vi "ReadConfigurationFile_Algo(old).vi"(0 "Default Configuration file path":path=path "C:/Users/GTron/Desktop/MOTHERSON v1.3/ZenGage V1.3.1/Configuration file/Algorithm Parameters Default.json", 5 "Override Configuration file path":path=path "C:/Users/GTron/Desktop/MOTHERSON v1.3/ZenGage V1.3.1/Configuration file/Algorithm Parameters Override.json", 7 "OutputClusterIn":T1={"Acknowledgement"={"Enqueuer"=refnum, "VIReference"=refnum, "VIName"=""}, "AllPartInfo"=[{"PartName"="", "NumberOfRacks"=0, "MeasurementIDsArray"=[], "MeasurementNamesArray"=[], "SpecValuesArray"=[]}], "PartInfo"={"PartName"="", "TotalCount"=0, "ReelCount"=0, "NumberOfRacks"=0, "MeasurementIDsArray"=[], "MeasurementNamesArray"=[], "SpecValuesArray"=[]}, "Result Cluster"={"Measurement Names Array"=[], "Pass-Fail Array"=[], "Measurement Values Array "=[], "Roi for overlay (Arrows) Array"=[], "Algo Type Array"=[], "Image Array"=[], "Clamp operations"=enum."Average Clamp", "  Search Direction "=[], "Images_Array_in"=[], "ResultPF"=FALSE, "Total Cluster Values"={"Total Fail"=0, "Total Pass"=0, "Total Count"=0}, "Reel Counter Cluster"={"Reel Fail"=0, "Reel Pass"=0, "Reel Count"=0}, "Tolerance  Array"=[], "Array of Cam Spec Control Bool"=[], "Control Pass Fail Array"=[], "Specification Pass Fail Array"=[], "Overlay Arrow Lines"=[], "Camera ID"=[], "Trigger count"=0, "Specification fail?"=FALSE}}, 9 "AlgoParameters":T6, 11 "error in":errorcluster) -> (4 "OutputClusterOut":T1={"Acknowledgement"={"Enqueuer"=refnum, "VIReference"=refnum, "VIName"=""}, "AllPartInfo"=[], "PartInfo"={"PartName"="", "TotalCount"=0, "ReelCount"=0, "NumberOfRacks"=0, "MeasurementIDsArray"=[], "MeasurementNamesArray"=[], "SpecValuesArray"=[]}, "Result Cluster"={"Measurement Names Array"=[], "Pass-Fail Array"=[], "Measurement Values Array "=[], "Roi for overlay (Arrows) Array"=[], "Algo Type Array"=[], "Image Array"=[], "Clamp operations"=enum."Average Clamp", "  Search Direction "=[], "Images_Array_in"=[], "ResultPF"=FALSE, "Total Cluster Values"={"Total Fail"=0, "Total Pass"=0, "Total Count"=0}, "Reel Counter Cluster"={"Reel Fail"=0, "Reel Pass"=0, "Reel Count"=0}, "Tolerance  Array"=[], "Array of Cam Spec Control Bool"=[], "Control Pass Fail Array"=[], "Specification Pass Fail Array"=[], "Overlay Arrow Lines"=[], "Camera ID"=[], "Trigger count"=0, "Specification fail?"=FALSE}}, 6 "AllAlgoParameters":T6, 15 "error out":errorcluster)   [LabVIEW 2015, in "Algorithm.lvclass"]
uses:
  FrameworkOverrides/Algorithm.lvclass
  Controls/OutputCluster.ctl
  <vilib>/ActorFramework/Message Enqueuer/Message Enqueuer.lvclass
  Common/Controls/Acknowledgement.ctl
  Common/Controls/AllPartInfo.ctl
  Controls/Result Cluster.ctl
panel:
  out "Queried Cluster":variant
  out "Default JSON string":string
  out "Override JSON string":string
  out "Error Message":string
  out "Output Merged Cluster":variant
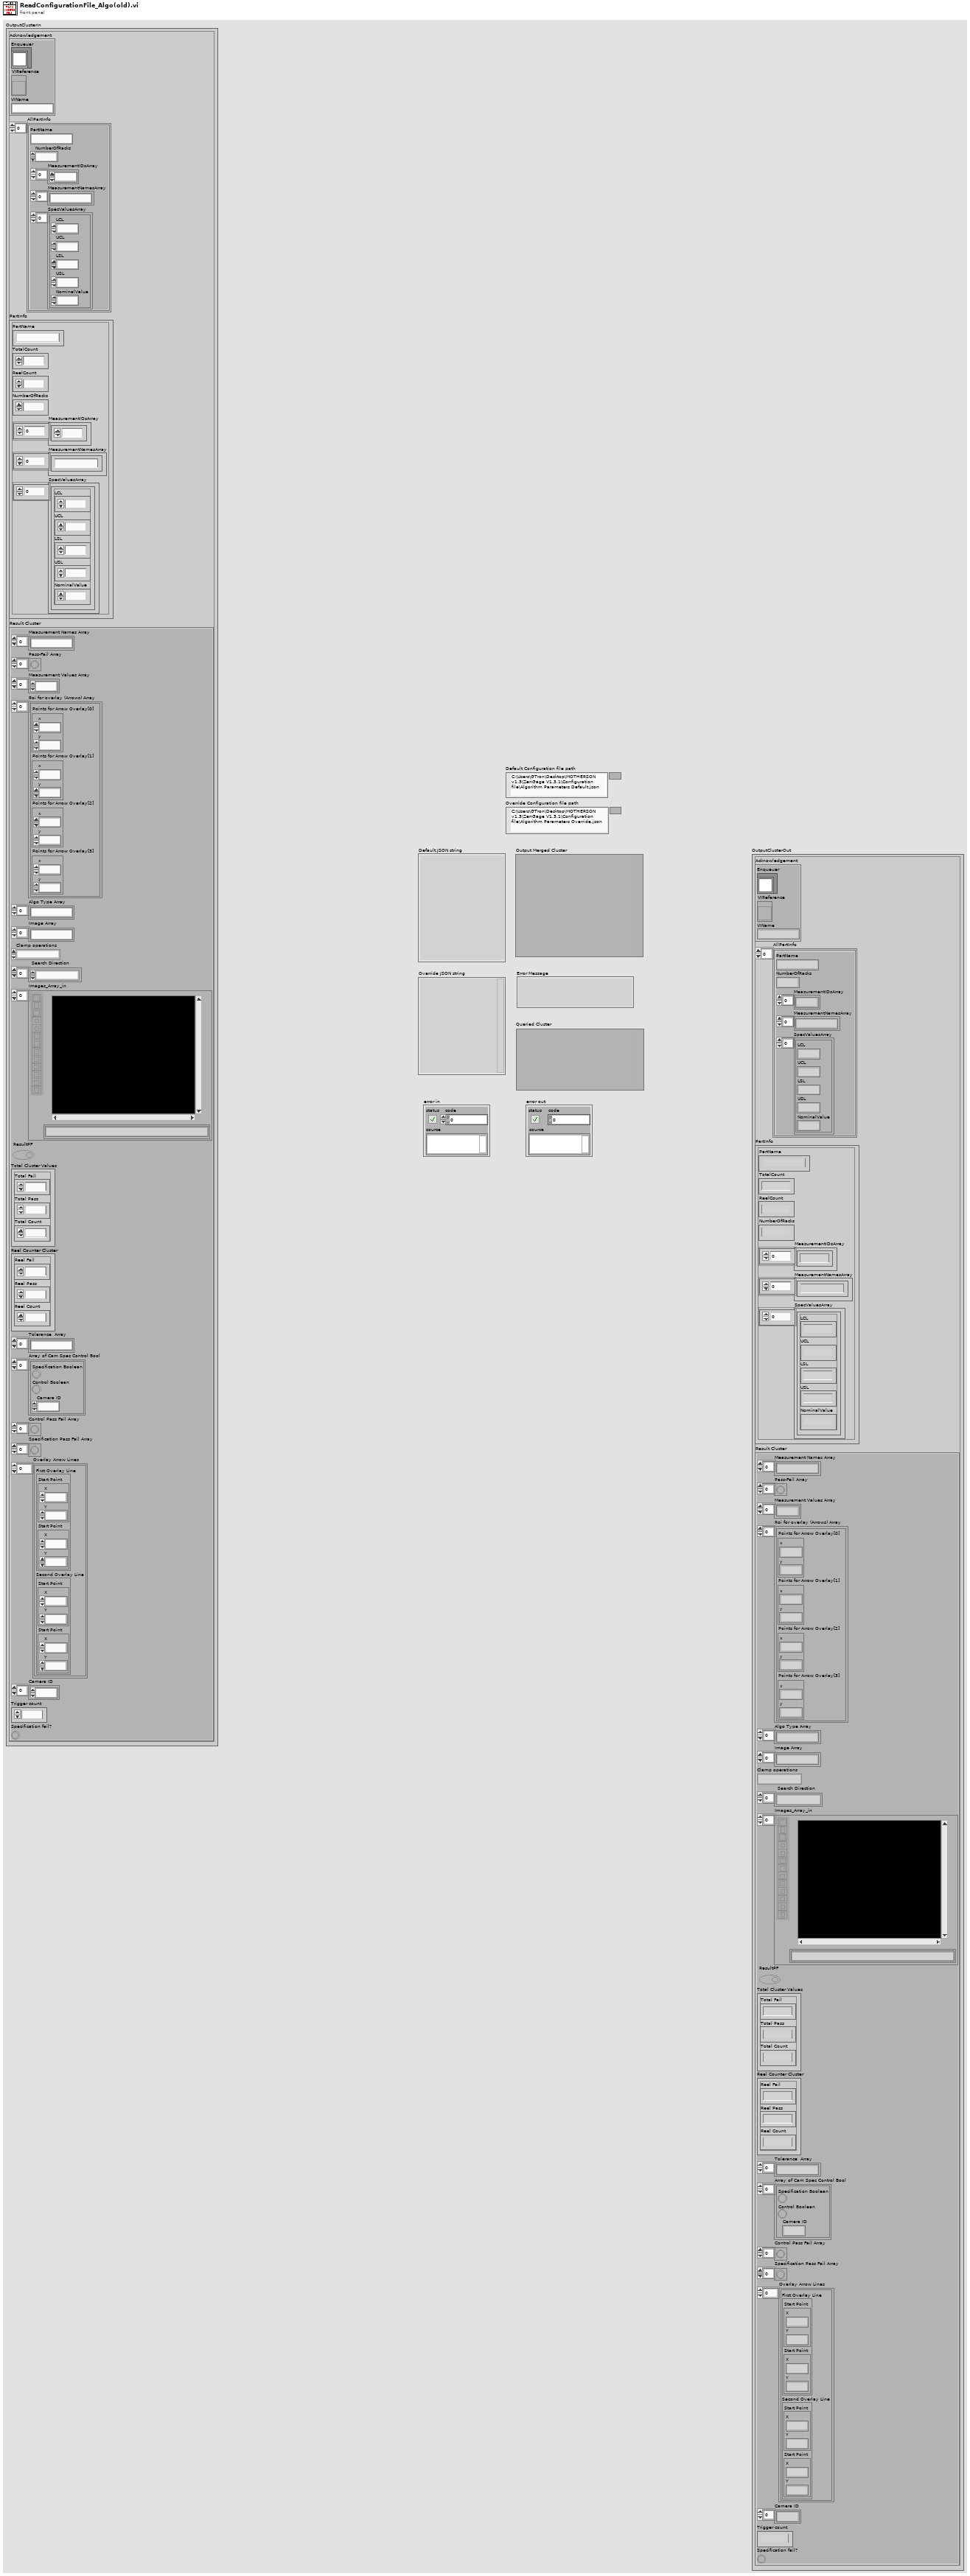
[diagram p1: front panel]
types:
  T1 = typedef "Algorithm.lvclass/OutputCluster.ctl" = cluster{"Acknowledgement":T2, "AllPartInfo":T3, "PartInfo":cluster{"PartName":string, "TotalCount":u64, "ReelCount":u64, "NumberOfRacks":u8, "MeasurementIDsArray":u16[], "MeasurementNamesArray":string[], "SpecValuesArray":cluster{"LCL":dbl, "UCL":dbl, "LSL":dbl, "USL":dbl, "NominalValue":dbl}[]}, "Result Cluster":T4}
  T2 = typedef "Acknowledgement.ctl" = cluster{"Enqueuer":refnum<class "Message Enqueuer.lvclass">, "VIReference":refnum<vi>, "VIName":string}
  T3 = typedef "AllPartInfo.ctl" = cluster{"PartName":string, "NumberOfRacks":u8, "MeasurementIDsArray":u16[], "MeasurementNamesArray":string[], "SpecValuesArray":cluster{"LCL":dbl, "UCL":dbl, "LSL":dbl, "USL":dbl, "NominalValue":dbl}[]}[]
  T4 = typedef "Algorithm.lvclass/Result Cluster.ctl" = cluster{"Measurement Names Array":string[], "Pass-Fail Array":bool[], "Measurement Values Array ":dbl[], "Roi for overlay (Arrows) Array":cluster{"Points for Arrow Overlay[0]":cluster{"x":dbl, "y":dbl}, "Points for Arrow Overlay[1]":cluster{"x":dbl, "y":dbl}, "Points for Arrow Overlay[2]":cluster{"x":dbl, "y":dbl}, "Points for Arrow Overlay[3]":cluster{"x":dbl, "y":dbl}}[], "Algo Type Array":string[], "Image Array":string[], "Clamp operations":enum16{"Min Clamp", "Max Clamp", "Average Clamp"}, "  Search Direction ":enum16{"Left to Right", "Right to Left", "Top to Bottom", "Bottom to Top"}[], "Images_Array_in":T5[], "ResultPF":bool, "Total Cluster Values":cluster{"Total Fail":u64, "Total Pass":u64, "Total Count":u64}, "Reel Counter Cluster":cluster{"Reel Fail":u64, "Reel Pass":u64, "Reel Count":u64}, "Tolerance  Array":string[], "Array of Cam Spec Control Bool":cluster{"Specification Boolean":bool, "Control Boolean":bool, "Camera ID":i8}[], "Control Pass Fail Array":bool[], "Specification Pass Fail Array":bool[], "Overlay Arrow Lines":cluster{"First Overlay Line ":cluster{"Start Point":cluster{"X":sgl, "Y":sgl}, "Start Point":cluster{"X":sgl, "Y":sgl}}, "Second Overlay Line ":cluster{"Start Point":cluster{"X":sgl, "Y":sgl}, "Start Point":cluster{"X":sgl, "Y":sgl}}}[], "Camera ID":i8[], "Trigger count":i32, "Specification fail?":bool}
  T5 = typedef "IMAQ Image.ctl" = refnum<image>
  T6 = cluster{"PartsList":cluster{"Name":string, "ImageStreams":cluster{"ThreadName":string, "RackEnable":bool, "ThreadId":i32, "RackId":i32, "DifferenceParameter":i32, "SplitCameraIDs":i32[], "ImagingViews":cluster{"ViewName":string, "ViewEnable":bool, "ImageID":i32, "CameraID":i32, "CalibrationFilePath":string, "CalibImageFormat":string, "ReferenceCoordSystem":cluster{"Method":cluster{"Algo":string, "BaseReference":cluster{"OriginX":i32, "OriginY":i32, "Angle":dbl, "AxisReference":i32}}, "ROI1":cluster{"ROI":cluster{"Left":i32, "Top":i32, "Right":i32, "Bottom":i32, "Rotation":dbl}, "EdgeOptions":cluster{"EdgePolarity":i32, "KernelSize":i32, "Width":i32, "MinimumEdgeStrength":i32, "InterpolationType":i32, "DataProcessingMethod":i32}, "LineOptions":cluster{"NumberofLines":i32, "Type":i32, "MinScore":i32, "MaxScore":i32, "Orientation":i32, "AngleRange":i32, "AngleTolerance":i32, "StepSize":i32, "MinSNR":i32, "MinPoints":i32, "HoughIterations":i32}, "Process":i32, "StepSize":i32, "SearchDirection":i32, "CircleEdgeOptions":cluster{"SearchDirection":i32, "EdgeOptions":cluster{"EdgePolarity":i32, "KernelSize":i32, "Width":i32, "MinimumEdgeStrength":i32, "InterpolationType":i32, "DataProcessingMethod":i32}}, "CircleFitOptions":cluster{"Process":i32, "StepSize":i32, "MAxPixelRadius":i32}, "CircleSearchDirection":i32, "CurveParameters":cluster{"ExtractionMode":i32, "EdgeThreshold":i32, "EdgeFilterSize":i32, "MinLength":i32, "RowSearchStepSize":i32, "ColSearchStepSize":i32, "MaxEndpointGap":i32, "Closed":bool, "Subpixel":bool}, "MinimumMatchScore":i32, "CircleDescriptor":cluster{"MinRadius":i32, "MaxRadius":i32}, "EllipseDescriptor":cluster{"MinMajorRadius":i32, "MaxMajorRadius":i32, "MinMinorRadius":i32, "MaxMinorRadius":i32}, "ParallelLines":cluster{"First":i32, "Second":i32, "Third":i32}}[], "Name":string, "OverlayOptions":cluster{"OverlayEnable":bool, "OverlayText":string, "OverlayCoords":i32[], "OverlayAngle":i32, "OverlayTextSize":i32, "OverlayTextColor":string, "OverlayROI":bool, "OverlayRakeLine":bool, "OverlayPoints":bool}}, "CameraAngle":dbl[]}[]}[], "Measurements":cluster{"RackID":i32, "ImageID":i32, "CameraID":i32, "MeasurementId":i32, "Name":string, "AlgoName":string, "Type":string, "MeasurementEnable":bool, "AlgorithmSequence":cluster{"RefernceEdge":cluster{"Enable":bool, "Method":string, "RefROI":cluster{"Left":i32, "Top":i32, "Right":i32, "Bottom":i32, "Rotation":dbl}, "EdgeOptions":cluster{"EdgePoarity":i32, "KernelSize":i32, "Width":i32, "MinimumEdgeStrength":i32, "InterpolationType":i32, "DataProcessingMethod":i32}, "LineOptions":cluster{"NumberofLines":i32, "Type":i32, "MinScore":i32, "MaxScore":i32, "Orientation":i32, "AngleRange":i32, "AngleTolerance":i32, "StepSize":i32, "MinSNR":i32, "MinPoints":i32, "HoughIterations":i32}, "SearchDirection":i32}, "Measurement":cluster{"ROI1":cluster{"Enable":bool, "ROI":cluster{"Left":i32, "Top":i32, "Right":i32, "Bottom":i32, "Rotation":dbl}, "EdgeOptions":cluster{"EdgePoarity":i32, "KernelSize":i32, "Width":i32, "MinimumEdgeStrength":i32, "InterpolationType":i32, "DataProcessingMethod":i32}, "LineOptions":cluster{"NumberofLines":i32, "Type":i32, "MinScore":i32, "MaxScore":i32, "Orientation":i32, "AngleRange":i32, "AngleTolerance":i32, "StepSize":i32, "MinSNR":i32, "MinPoints":i32, "HoughIterations":i32}, "Process":i32, "StepSize":i32, "SearchDirection":i32, "CircleEdgeOptions":cluster{"SearchDirection":i32, "EdgeOptions":cluster{"EdgePoarity":i32, "KernelSize":i32, "Width":i32, "MinimumEdgeStrength":i32, "InterpolationType":i32, "DataProcessingMethod":i32}}, "CircleFitOptions":cluster{"Process":i32, "StepSize":i32, "MAxPixelRadius":dbl}, "CircleSearchDirection":i32, "CurveParameters":cluster{"ExtractionMode":i32, "EdgeThreshold":i32, "EdgeFilterSize":i32, "MinLength":i32, "RowSearchStepSize":i32, "ColSearchStepSize":i32, "MaxEndpointGap":i32, "Closed":bool, "Subpixel":bool}, "MinimumMatchScore":i32, "CircleDescriptor":cluster{"MinRadius":i32, "MaxRadius":i32}, "EllipseDescriptor":cluster{"MinMajorRadius":i32, "MaxMajorRadius":i32, "MinMinorRadius":i32, "MaxMinorRadius":i32}}, "ROI2":cluster{"Enable":bool, "ROI":cluster{"Left":i32, "Top":i32, "Right":i32, "Bottom":i32, "Rotation":dbl}, "EdgeOptions":cluster{"EdgePoarity":i32, "KernelSize":i32, "Width":i32, "MinimumEdgeStrength":i32, "InterpolationType":i32, "DataProcessingMethod":i32}, "LineOptions":cluster{"NumberofLines":i32, "Type":i32, "MinScore":i32, "MaxScore":i32, "Orientation":i32, "AngleRange":i32, "AngleTolerance":i32, "StepSize":i32, "MinSNR":i32, "MinPoints":i32, "HoughIterations":i32}, "Process":i32, "StepSize":i32, "SearchDirection":i32, "CircleEdgeOptions":cluster{"SearchDirection":i32, "EdgeOptions":cluster{"EdgePoarity":i32, "KernelSize":i32, "Width":i32, "MinimumEdgeStrength":i32, "InterpolationType":i32, "DataProcessingMethod":i32}}, "CircleFitOptions":cluster{"Process":i32, "StepSize":i32, "MAxPixelRadius":dbl}, "CircleSearchDirection":i32, "CurveParameters":cluster{"ExtractionMode":i32, "EdgeThreshold":i32, "EdgeFilterSize":i32, "MinLength":i32, "RowSearchStepSize":i32, "ColSearchStepSize":i32, "MaxEndpointGap":i32, "Closed":bool, "Subpixel":bool}, "MinimumMatchScore":i32, "CircleDescriptor":cluster{"MinRadius":i32, "MaxRadius":i32}, "EllipseDescriptor":cluster{"MinMajorRadius":i32, "MaxMajorRadius":i32, "MinMinorRadius":i32, "MaxMinorRadius":i32}}}}, "MathExpression":cluster{"Algorithm":string, "MathExpression":string, "ResultVariable":string}, "MathCorrectionParameters":cluster{"Radius":dbl, "CurlGap":dbl, "Thickness":dbl, "MeasurementIndices":i32[], "MathAlgoName":string, "MathAlgoFormula":string, "CorrectionForAngle":i32[], "NumericAray":i32[], "StringArray":string[]}, "ResultVariableCluster":cluster{"RVName":string, "RVSequence":string, "RVIndex":i32, "RVID":i32, "RVValue":dbl}, "CalibrationCoefficients":cluster{"A1":dbl, "A2":dbl, "A3":dbl}, "UserCalibCoefficients":cluster{"UserCorrectionLinearityCoeff":dbl, "UserCorrectionBiasCoeff":dbl}, "SpecValues":cluster{"LCL":dbl, "UCL":dbl, "LSL":dbl, "USL":dbl, "NominalValue":dbl}, "OverlayOptions":cluster{"OverlayEnable":bool, "OverlayText":string, "OverlayCoords":i32[], "OverlayAngle":i32, "OverlayTextSize":i32, "OverlayTextColor":string, "OverlayROI":bool, "OverlayRakeLine":bool, "OverlayPoints":bool}, "DatalogEnable":bool, "DisplayIcon":string}[]}[]}
  T7 = cluster{"Name":string, "ImageStreams":cluster{"ThreadName":string, "RackEnable":bool, "ThreadId":i32, "RackId":i32, "DifferenceParameter":i32, "SplitCameraIDs":i32[], "ImagingViews":cluster{"ViewName":string, "ViewEnable":bool, "ImageID":i32, "CameraID":i32, "CalibrationFilePath":string, "CalibImageFormat":string, "ReferenceCoordSystem":cluster{"Method":cluster{"Algo":string, "BaseReference":cluster{"OriginX":i32, "OriginY":i32, "Angle":dbl, "AxisReference":i32}}, "ROI1":cluster{"ROI":cluster{"Left":i32, "Top":i32, "Right":i32, "Bottom":i32, "Rotation":dbl}, "EdgeOptions":cluster{"EdgePolarity":i32, "KernelSize":i32, "Width":i32, "MinimumEdgeStrength":i32, "InterpolationType":i32, "DataProcessingMethod":i32}, "LineOptions":cluster{"NumberofLines":i32, "Type":i32, "MinScore":i32, "MaxScore":i32, "Orientation":i32, "AngleRange":i32, "AngleTolerance":i32, "StepSize":i32, "MinSNR":i32, "MinPoints":i32, "HoughIterations":i32}, "Process":i32, "StepSize":i32, "SearchDirection":i32, "CircleEdgeOptions":cluster{"SearchDirection":i32, "EdgeOptions":cluster{"EdgePolarity":i32, "KernelSize":i32, "Width":i32, "MinimumEdgeStrength":i32, "InterpolationType":i32, "DataProcessingMethod":i32}}, "CircleFitOptions":cluster{"Process":i32, "StepSize":i32, "MAxPixelRadius":i32}, "CircleSearchDirection":i32, "CurveParameters":cluster{"ExtractionMode":i32, "EdgeThreshold":i32, "EdgeFilterSize":i32, "MinLength":i32, "RowSearchStepSize":i32, "ColSearchStepSize":i32, "MaxEndpointGap":i32, "Closed":bool, "Subpixel":bool}, "MinimumMatchScore":i32, "CircleDescriptor":cluster{"MinRadius":i32, "MaxRadius":i32}, "EllipseDescriptor":cluster{"MinMajorRadius":i32, "MaxMajorRadius":i32, "MinMinorRadius":i32, "MaxMinorRadius":i32}, "ParallelLines":cluster{"First":i32, "Second":i32, "Third":i32}}[], "Name":string, "OverlayOptions":cluster{"OverlayEnable":bool, "OverlayText":string, "OverlayCoords":i32[], "OverlayAngle":i32, "OverlayTextSize":i32, "OverlayTextColor":string, "OverlayROI":bool, "OverlayRakeLine":bool, "OverlayPoints":bool}}, "CameraAngle":dbl[]}[]}[], "Measurements":cluster{"RackID":i32, "ImageID":i32, "CameraID":i32, "MeasurementId":i32, "Name":string, "AlgoName":string, "Type":string, "MeasurementEnable":bool, "AlgorithmSequence":cluster{"RefernceEdge":cluster{"Enable":bool, "Method":string, "RefROI":cluster{"Left":i32, "Top":i32, "Right":i32, "Bottom":i32, "Rotation":dbl}, "EdgeOptions":cluster{"EdgePoarity":i32, "KernelSize":i32, "Width":i32, "MinimumEdgeStrength":i32, "InterpolationType":i32, "DataProcessingMethod":i32}, "LineOptions":cluster{"NumberofLines":i32, "Type":i32, "MinScore":i32, "MaxScore":i32, "Orientation":i32, "AngleRange":i32, "AngleTolerance":i32, "StepSize":i32, "MinSNR":i32, "MinPoints":i32, "HoughIterations":i32}, "SearchDirection":i32}, "Measurement":cluster{"ROI1":cluster{"Enable":bool, "ROI":cluster{"Left":i32, "Top":i32, "Right":i32, "Bottom":i32, "Rotation":dbl}, "EdgeOptions":cluster{"EdgePoarity":i32, "KernelSize":i32, "Width":i32, "MinimumEdgeStrength":i32, "InterpolationType":i32, "DataProcessingMethod":i32}, "LineOptions":cluster{"NumberofLines":i32, "Type":i32, "MinScore":i32, "MaxScore":i32, "Orientation":i32, "AngleRange":i32, "AngleTolerance":i32, "StepSize":i32, "MinSNR":i32, "MinPoints":i32, "HoughIterations":i32}, "Process":i32, "StepSize":i32, "SearchDirection":i32, "CircleEdgeOptions":cluster{"SearchDirection":i32, "EdgeOptions":cluster{"EdgePoarity":i32, "KernelSize":i32, "Width":i32, "MinimumEdgeStrength":i32, "InterpolationType":i32, "DataProcessingMethod":i32}}, "CircleFitOptions":cluster{"Process":i32, "StepSize":i32, "MAxPixelRadius":dbl}, "CircleSearchDirection":i32, "CurveParameters":cluster{"ExtractionMode":i32, "EdgeThreshold":i32, "EdgeFilterSize":i32, "MinLength":i32, "RowSearchStepSize":i32, "ColSearchStepSize":i32, "MaxEndpointGap":i32, "Closed":bool, "Subpixel":bool}, "MinimumMatchScore":i32, "CircleDescriptor":cluster{"MinRadius":i32, "MaxRadius":i32}, "EllipseDescriptor":cluster{"MinMajorRadius":i32, "MaxMajorRadius":i32, "MinMinorRadius":i32, "MaxMinorRadius":i32}}, "ROI2":cluster{"Enable":bool, "ROI":cluster{"Left":i32, "Top":i32, "Right":i32, "Bottom":i32, "Rotation":dbl}, "EdgeOptions":cluster{"EdgePoarity":i32, "KernelSize":i32, "Width":i32, "MinimumEdgeStrength":i32, "InterpolationType":i32, "DataProcessingMethod":i32}, "LineOptions":cluster{"NumberofLines":i32, "Type":i32, "MinScore":i32, "MaxScore":i32, "Orientation":i32, "AngleRange":i32, "AngleTolerance":i32, "StepSize":i32, "MinSNR":i32, "MinPoints":i32, "HoughIterations":i32}, "Process":i32, "StepSize":i32, "SearchDirection":i32, "CircleEdgeOptions":cluster{"SearchDirection":i32, "EdgeOptions":cluster{"EdgePoarity":i32, "KernelSize":i32, "Width":i32, "MinimumEdgeStrength":i32, "InterpolationType":i32, "DataProcessingMethod":i32}}, "CircleFitOptions":cluster{"Process":i32, "StepSize":i32, "MAxPixelRadius":dbl}, "CircleSearchDirection":i32, "CurveParameters":cluster{"ExtractionMode":i32, "EdgeThreshold":i32, "EdgeFilterSize":i32, "MinLength":i32, "RowSearchStepSize":i32, "ColSearchStepSize":i32, "MaxEndpointGap":i32, "Closed":bool, "Subpixel":bool}, "MinimumMatchScore":i32, "CircleDescriptor":cluster{"MinRadius":i32, "MaxRadius":i32}, "EllipseDescriptor":cluster{"MinMajorRadius":i32, "MaxMajorRadius":i32, "MinMinorRadius":i32, "MaxMinorRadius":i32}}}}, "MathExpression":cluster{"Algorithm":string, "MathExpression":string, "ResultVariable":string}, "MathCorrectionParameters":cluster{"Radius":dbl, "CurlGap":dbl, "Thickness":dbl, "MeasurementIndices":i32[], "MathAlgoName":string, "MathAlgoFormula":string, "CorrectionForAngle":i32[], "NumericAray":i32[], "StringArray":string[]}, "ResultVariableCluster":cluster{"RVName":string, "RVSequence":string, "RVIndex":i32, "RVID":i32, "RVValue":dbl}, "CalibrationCoefficients":cluster{"A1":dbl, "A2":dbl, "A3":dbl}, "UserCalibCoefficients":cluster{"UserCorrectionLinearityCoeff":dbl, "UserCorrectionBiasCoeff":dbl}, "SpecValues":cluster{"LCL":dbl, "UCL":dbl, "LSL":dbl, "USL":dbl, "NominalValue":dbl}, "OverlayOptions":cluster{"OverlayEnable":bool, "OverlayText":string, "OverlayCoords":i32[], "OverlayAngle":i32, "OverlayTextSize":i32, "OverlayTextColor":string, "OverlayROI":bool, "OverlayRakeLine":bool, "OverlayPoints":bool}, "DatalogEnable":bool, "DisplayIcon":string}[]}[]
  T8 = cluster{"PartName":string, "NumberOfRacks":u8, "MeasurementIDsArray":u16[], "MeasurementNamesArray":string[], "SpecValuesArray":cluster{"LCL":dbl, "UCL":dbl, "LSL":dbl, "USL":dbl, "NominalValue":dbl}[]}
  T9 = cluster{"PartName":string, "NumberOfRacks":u8, "MeasurementIDsArray":u16[], "MeasurementNamesArray":string[], "SpecValuesArray":cluster{"LCL":dbl, "UCL":dbl, "LSL":dbl, "USL":dbl, "NominalValue":dbl}[]}[]
  T10 = cluster{"RackID":i32, "ImageID":i32, "CameraID":i32, "MeasurementId":i32, "Name":string, "AlgoName":string, "Type":string, "MeasurementEnable":bool, "AlgorithmSequence":cluster{"RefernceEdge":cluster{"Enable":bool, "Method":string, "RefROI":cluster{"Left":i32, "Top":i32, "Right":i32, "Bottom":i32, "Rotation":dbl}, "EdgeOptions":cluster{"EdgePoarity":i32, "KernelSize":i32, "Width":i32, "MinimumEdgeStrength":i32, "InterpolationType":i32, "DataProcessingMethod":i32}, "LineOptions":cluster{"NumberofLines":i32, "Type":i32, "MinScore":i32, "MaxScore":i32, "Orientation":i32, "AngleRange":i32, "AngleTolerance":i32, "StepSize":i32, "MinSNR":i32, "MinPoints":i32, "HoughIterations":i32}, "SearchDirection":i32}, "Measurement":cluster{"ROI1":cluster{"Enable":bool, "ROI":cluster{"Left":i32, "Top":i32, "Right":i32, "Bottom":i32, "Rotation":dbl}, "EdgeOptions":cluster{"EdgePoarity":i32, "KernelSize":i32, "Width":i32, "MinimumEdgeStrength":i32, "InterpolationType":i32, "DataProcessingMethod":i32}, "LineOptions":cluster{"NumberofLines":i32, "Type":i32, "MinScore":i32, "MaxScore":i32, "Orientation":i32, "AngleRange":i32, "AngleTolerance":i32, "StepSize":i32, "MinSNR":i32, "MinPoints":i32, "HoughIterations":i32}, "Process":i32, "StepSize":i32, "SearchDirection":i32, "CircleEdgeOptions":cluster{"SearchDirection":i32, "EdgeOptions":cluster{"EdgePoarity":i32, "KernelSize":i32, "Width":i32, "MinimumEdgeStrength":i32, "InterpolationType":i32, "DataProcessingMethod":i32}}, "CircleFitOptions":cluster{"Process":i32, "StepSize":i32, "MAxPixelRadius":dbl}, "CircleSearchDirection":i32, "CurveParameters":cluster{"ExtractionMode":i32, "EdgeThreshold":i32, "EdgeFilterSize":i32, "MinLength":i32, "RowSearchStepSize":i32, "ColSearchStepSize":i32, "MaxEndpointGap":i32, "Closed":bool, "Subpixel":bool}, "MinimumMatchScore":i32, "CircleDescriptor":cluster{"MinRadius":i32, "MaxRadius":i32}, "EllipseDescriptor":cluster{"MinMajorRadius":i32, "MaxMajorRadius":i32, "MinMinorRadius":i32, "MaxMinorRadius":i32}}, "ROI2":cluster{"Enable":bool, "ROI":cluster{"Left":i32, "Top":i32, "Right":i32, "Bottom":i32, "Rotation":dbl}, "EdgeOptions":cluster{"EdgePoarity":i32, "KernelSize":i32, "Width":i32, "MinimumEdgeStrength":i32, "InterpolationType":i32, "DataProcessingMethod":i32}, "LineOptions":cluster{"NumberofLines":i32, "Type":i32, "MinScore":i32, "MaxScore":i32, "Orientation":i32, "AngleRange":i32, "AngleTolerance":i32, "StepSize":i32, "MinSNR":i32, "MinPoints":i32, "HoughIterations":i32}, "Process":i32, "StepSize":i32, "SearchDirection":i32, "CircleEdgeOptions":cluster{"SearchDirection":i32, "EdgeOptions":cluster{"EdgePoarity":i32, "KernelSize":i32, "Width":i32, "MinimumEdgeStrength":i32, "InterpolationType":i32, "DataProcessingMethod":i32}}, "CircleFitOptions":cluster{"Process":i32, "StepSize":i32, "MAxPixelRadius":dbl}, "CircleSearchDirection":i32, "CurveParameters":cluster{"ExtractionMode":i32, "EdgeThreshold":i32, "EdgeFilterSize":i32, "MinLength":i32, "RowSearchStepSize":i32, "ColSearchStepSize":i32, "MaxEndpointGap":i32, "Closed":bool, "Subpixel":bool}, "MinimumMatchScore":i32, "CircleDescriptor":cluster{"MinRadius":i32, "MaxRadius":i32}, "EllipseDescriptor":cluster{"MinMajorRadius":i32, "MaxMajorRadius":i32, "MinMinorRadius":i32, "MaxMinorRadius":i32}}}}, "MathExpression":cluster{"Algorithm":string, "MathExpression":string, "ResultVariable":string}, "MathCorrectionParameters":cluster{"Radius":dbl, "CurlGap":dbl, "Thickness":dbl, "MeasurementIndices":i32[], "MathAlgoName":string, "MathAlgoFormula":string, "CorrectionForAngle":i32[], "NumericAray":i32[], "StringArray":string[]}, "ResultVariableCluster":cluster{"RVName":string, "RVSequence":string, "RVIndex":i32, "RVID":i32, "RVValue":dbl}, "CalibrationCoefficients":cluster{"A1":dbl, "A2":dbl, "A3":dbl}, "UserCalibCoefficients":cluster{"UserCorrectionLinearityCoeff":dbl, "UserCorrectionBiasCoeff":dbl}, "SpecValues":cluster{"LCL":dbl, "UCL":dbl, "LSL":dbl, "USL":dbl, "NominalValue":dbl}, "OverlayOptions":cluster{"OverlayEnable":bool, "OverlayText":string, "OverlayCoords":i32[], "OverlayAngle":i32, "OverlayTextSize":i32, "OverlayTextColor":string, "OverlayROI":bool, "OverlayRakeLine":bool, "OverlayPoints":bool}, "DatalogEnable":bool, "DisplayIcon":string}[]
  T11 = cluster{"LCL":dbl, "UCL":dbl, "LSL":dbl, "USL":dbl, "NominalValue":dbl}
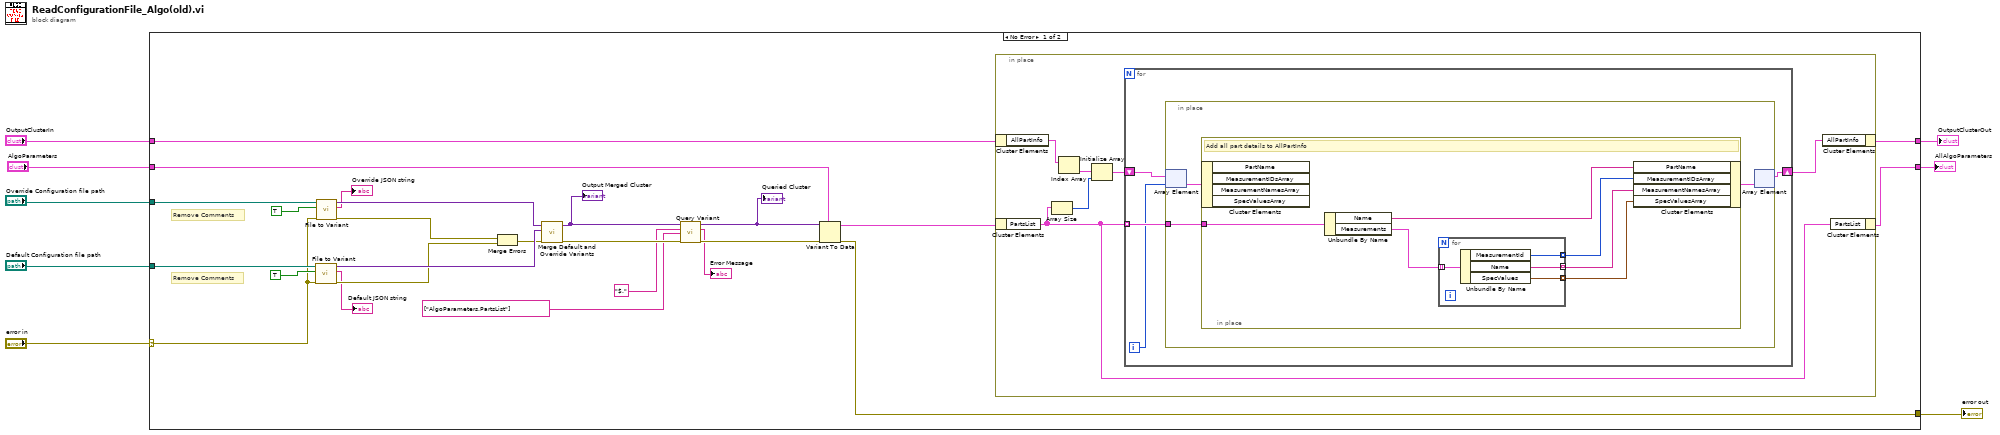
[diagram p0: block diagram]
diagram:
  n1 = case shown="No Error" "error in" {
    selector: "error in" -> [w18 w58]
    tunnel: "Override Configuration file path" -> [w31 _]
    tunnel: "Default Configuration file path" -> [w30 _]
    tunnel: [w24 w58] -> w6
    tunnel: "OutputClusterIn" -> [w17 w59]
    tunnel: [w16 w59] -> w1
    tunnel: "AlgoParameters" -> [w13 w57]
    tunnel: [w9 w57] -> w2
    frame No Error {
      # "Remove Comments"
      # "Remove Comments"
      n2 = call <vilib>:"File to Variant.vi"("JSON FilePath"=w30, "Remove Comments?"=TRUE, "error in (no error)"=w18) -> ("JSON Variant"=w28:variant, "Error message out"=→"Default JSON string":string, "error out"=w26:errorcluster)  [unwired: 4 in, 1 out]
      n3 = call <vilib>:"File to Variant.vi"("JSON FilePath"=w31, "Remove Comments?"=TRUE, "error in (no error)"=w18) -> ("JSON Variant"=w29:variant, "Error message out"=→"Override JSON string":string, "error out"=w25:errorcluster)  [unwired: 4 in, 1 out]
      n4 = Merge Errors(w25, w26) -> (w27:errorcluster)
      n5 = call <vilib>:"Merge Default and Override Variants.vi"("error in (no error)"=w27, "Default VCluster"=w28, "Override VCluster"=w29) -> ("error out"=w23:errorcluster, "Output Merged Cluster"=w15:variant)  [unwired: 7 in]
      "Output Merged Cluster" <- w15
      n6 = call <vilib>:"Query Variant.vi"("VCluster in"=w15, "basePath in"="$.", "pathList"=string[] ["AlgoParameters.PartsList"], "error IO"=w23) -> ("VCluster\n out"=w14:variant, "Error Message"=→"Error Message":string, "error out"=w22:errorcluster)  [unwired: 8 in, 1 out]
      "Queried Cluster" <- w14
      n7 = Variant To Data(error in=w22, type=w13, Variant=w14) -> (data=w10:T6, error out=w24:errorcluster)
      n8 = in-place {
        n9 = in-place-cluster #1(w17) -> ("AllPartInfo"=w38:T3)
        n10 = in-place-cluster #2(w10) -> ("PartsList"=w36:T7)
        n11 = Array Size(array=w36) -> (size(s)=w35:i32)
        n12 = Index Array(array=w38) -> (element=w37:T8)  [unwired: 1 in]
        n13 = Initialize Array(w37, w35) -> (w34:T9)
        n14 = for {
          tunnel: w36 -> [w43] mode=indexing
          shift-right: [w40] -> w39
          shift-left: w34 -> [w42]
          i -> [w41]
          n15 = in-place {
            in-place-border: w43 -> [w44]
            n16 = in-place-array #3(w42, w41) -> (w46:T8)
            n17 = in-place {
              in-place-border: w44 -> [w52]
              # "Add all part details to AllPartInfo"
              n18 = in-place-cluster #4(w46) -> ()  [unwired: 4 out]
              n19 = Unbundle By Name(w52) -> ("Name"=w48:string, "Measurements"=w51:T10)
              n20 = for {
                tunnel: w51 -> [w56] mode=indexing
                tunnel: [w55] -> w49 mode=indexing
                tunnel: [w54] -> w50 mode=indexing
                tunnel: [w53] -> w47 mode=indexing
                n21 = Unbundle By Name(w56) -> ("MeasurementId"=w55:i32, "Name"=w54:string, "SpecValues"=w53:T11)
              }
              n22 = in-place-cluster #4("PartName"=w48, "MeasurementIDsArray"=w49, "MeasurementNamesArray"=w50, "SpecValuesArray"=w47) -> (w45:T8)
            }
            n23 = in-place-array #3(w45) -> (w40:T9)  [unwired: 1 out]
          }
        }
        n24 = in-place-cluster #1("AllPartInfo"=w39) -> (w16:T1)
        n25 = in-place-cluster #2("PartsList"=w36) -> (w9:T6)
      }
    }
    frame Error {
    }
  }
  "OutputClusterOut" <- w1
  "AllAlgoParameters" <- w2
  "error out" <- w6
